vi "Bit_machine.vi"() -> ()   [LabVIEW 2019]
panel:
  in  "Operacja":T1(ring)
  out "C 8":bool
  out "C 7":bool
  out "C 6":bool
  out "C 5":bool
  out "C 4":bool
  out "C 3":bool
  out "C 2":bool
  out "C 1":bool
  in  "B 8":bool
  in  "B 7":bool
  in  "B 6":bool
  in  "B 5":bool
  in  "B 4":bool
  in  "B 3":bool
  in  "B 2":bool
  in  "B 1":bool
  in  "A 8":bool
  in  "A 7":bool
  in  "A 6":bool
  in  "A 5":bool
  in  "A 4":bool
  in  "A 3":bool
  in  "A 2":bool
  in  "A 1":bool
  in  "?":bool
  # "Bajt pierwszy"
  # "Bajt drugi"
  # "Wynik:"
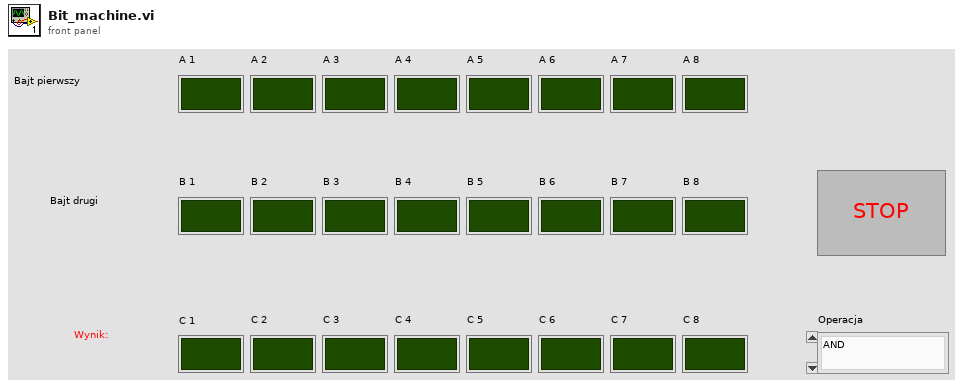
[diagram p1: front panel]
types:
  T1 = enum16{"AND", "OR", "XOR", "Not AND", "Not OR", "Not XOR", "Implies"}
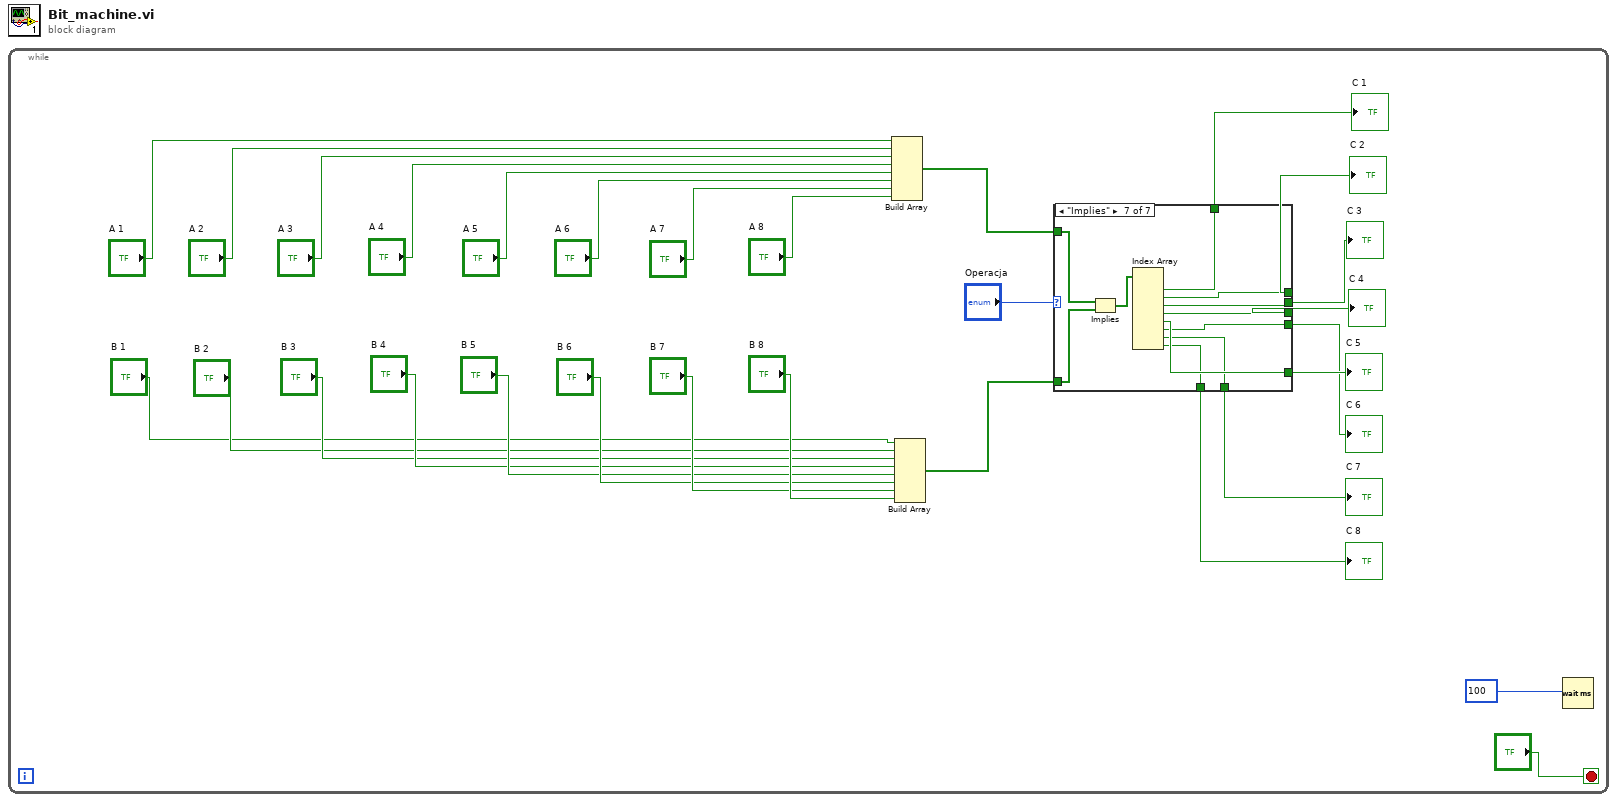
[diagram p0: block diagram]
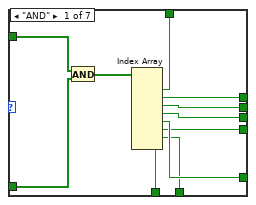
[diagram p2: hidden frame]
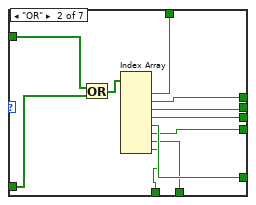
[diagram p3: hidden frame]
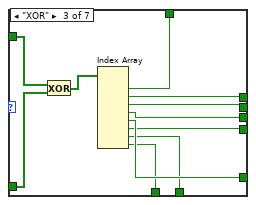
[diagram p4: hidden frame]
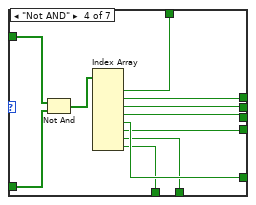
[diagram p5: hidden frame]
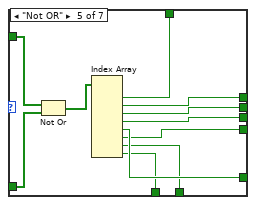
[diagram p6: hidden frame]
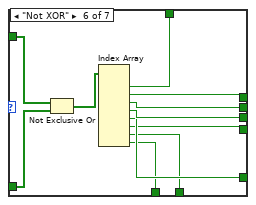
[diagram p7: hidden frame]
diagram:
  n1 = while {
    stop <- "?" stop-if-true
    n2 = Build Array("A 1", "A 2", "A 3", "A 4", "A 5", "A 6", "A 7", "A 8") -> (w12:bool[])
    n3 = Build Array("B 1", "B 2", "B 3", "B 4", "B 5", "B 6", "B 7", "B 8") -> (w11:bool[])
    n4 = case shown="\"Implies\"" "Operacja" {
      tunnel: w12 -> [w40 w51 w62 w73 w84 w95 w106]
      tunnel: w11 -> [w39 w50 w61 w72 w83 w94 w105]
      tunnel: [w37 w49 w59 w70 w81 w92 w103] -> w3
      tunnel: [w36 w46 w57 w68 w79 w90 w101] -> w10
      tunnel: [w35 w47 w58 w69 w80 w91 w102] -> w9
      tunnel: [w34 w45 w56 w67 w78 w89 w100] -> w8
      tunnel: [w33 w44 w55 w66 w77 w88 w99] -> w7
      tunnel: [w32 w43 w54 w65 w76 w87 w98] -> w6
      tunnel: [w31 w42 w53 w64 w75 w86 w97] -> w5
      tunnel: [w30 w41 w52 w63 w74 w85 w96] -> w4
      frame "AND" {
        n5 = And(x=w40, y=w39) -> (x .and. y?=w38:bool[])
        n6 = Index Array(array=w38) -> (element #1=w37:bool, element #2=w35:bool, element #3=w36:bool, element #4=w34:bool, element #5=w33:bool, element #6=w32:bool, element #7=w31:bool, element #8=w30:bool)  [unwired: 8 in]
      }
      frame "OR" {
        n7 = Or(x=w51, y=w50) -> (x .or. y?=w48:bool[])
        n8 = Index Array(array=w48) -> (element #1=w49:bool, element #2=w47:bool, element #3=w46:bool, element #4=w45:bool, element #5=w44:bool, element #6=w43:bool, element #7=w42:bool, element #8=w41:bool)  [unwired: 8 in]
      }
      frame "XOR" {
        n9 = Exclusive Or(1:w61, 2:w62) -> (0:w60:bool[])
        n10 = Index Array(array=w60) -> (element #1=w59:bool, element #2=w58:bool, element #3=w57:bool, element #4=w56:bool, element #5=w55:bool, element #6=w54:bool, element #7=w53:bool, element #8=w52:bool)  [unwired: 8 in]
      }
      frame "Not AND" {
        n11 = Not And(1:w72, 2:w73) -> (0:w71:bool[])
        n12 = Index Array(array=w71) -> (element #1=w70:bool, element #2=w69:bool, element #3=w68:bool, element #4=w67:bool, element #5=w66:bool, element #6=w65:bool, element #7=w64:bool, element #8=w63:bool)  [unwired: 8 in]
      }
      frame "Not OR" {
        n13 = Not Or(1:w83, 2:w84) -> (0:w82:bool[])
        n14 = Index Array(array=w82) -> (element #1=w81:bool, element #2=w80:bool, element #3=w79:bool, element #4=w78:bool, element #5=w77:bool, element #6=w76:bool, element #7=w75:bool, element #8=w74:bool)  [unwired: 8 in]
      }
      frame "Not XOR" {
        n15 = Not Exclusive Or(1:w94, 2:w95) -> (0:w93:bool[])
        n16 = Index Array(array=w93) -> (element #1=w92:bool, element #2=w91:bool, element #3=w90:bool, element #4=w89:bool, element #5=w88:bool, element #6=w87:bool, element #7=w86:bool, element #8=w85:bool)  [unwired: 8 in]
      }
      frame "Implies" {
        n17 = Implies(1:w105, 2:w106) -> (0:w104:bool[])
        n18 = Index Array(array=w104) -> (element #1=w103:bool, element #2=w102:bool, element #3=w101:bool, element #4=w100:bool, element #5=w99:bool, element #6=w98:bool, element #7=w97:bool, element #8=w96:bool)  [unwired: 8 in]
      }
    }
    "C 1" <- w3
    "C 2" <- w9
    "C 3" <- w10
    "C 4" <- w8
    "C 5" <- w7
    "C 6" <- w6
    "C 7" <- w5
    "C 8" <- w4
    n19 = Wait (ms)(milliseconds to wait=100) -> ()  [unwired: 1 out]
  }
